vi "Load New Value.vi"(7 "Reinit":bool, 8 "error in (no error)":errorcluster, 10 "New Value":i64, 11 "Stats_I64_CIF_U in":refnum<class "Stats_I64_CIF_U.lvclass">) -> (0 "error out":errorcluster, 3 "Stats_I64_CIF_U out":refnum<class "Stats_I64_CIF_U.lvclass">)   [LabVIEW 2021, in "Stats_CIF_U.lvlib" / "Stats_I64_CIF_U.lvclass"]
doc: "Load a new data value into the statistics class. This VI should be used when the value has been externally calculated."
uses:
  Stats_I64_CIF_U.lvclass
  Stats_I64_CIF_U.lvclass/Stats_I64_CIF_U.ctl
  dfabcf33-0dbc-4041-80a5-3dc0c86d2989.vi
  dfabcf33-0dbc-4041-80a5-3dc0c86d2989.vi/9eb60a9a-770f-4d2d-8b3f-8465c267ecc9.vi
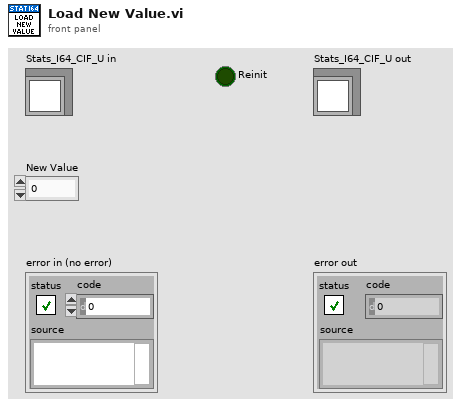
[diagram p1: front panel]
types:
  T1 = typedef "Stats_CIF_U.lvlib/I64 Stat Data.ctl" = cluster{"Last Value":i64, "Max":i64, "Min":i64, "Common ":T2}
  T2 = typedef "Stats_CIF_U.lvlib/Common Stat Data.ctl" = cluster{"Iteration":u32, "Max History":i32, "Average":dbl}
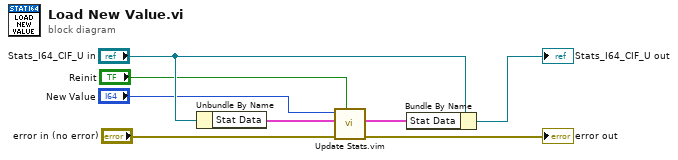
[diagram p0: block diagram]
diagram:
  n1 = Unbundle By Name("Stats_I64_CIF_U in") -> ("Stat Data"=w6:T1)
  n2 = call "Update Stats.vim"("Reinit"="Reinit", "error in"="error in (no error)", "Stat Data In"=w6, "New Value"="New Value") -> ("error out"=→"error out":errorcluster, "Stat Data Out"=w5:T1)  [unwired: 6 in]
  n3 = Bundle By Name(cluster="Stats_I64_CIF_U in", "Stat Data"=w5) -> (→"Stats_I64_CIF_U out":refnum<class "Stats_I64_CIF_U.lvclass">)
